vi "AlliGator Plot Histogram Event.vi"(8 "Error In":errorcluster, 11 "Mouse Click Event Data":T1) -> (0 "Error Out":errorcluster, 1 "Message":string)   [LabVIEW 2021, in "AlliGator Lifetime & Other Parameters.lvlib"]
uses:
  AlliGator Lifetime & Other Parameters.lvlib
  Graphs/XY Graph/XY Graph Mouse Click Event Data.ctl
  Graphs/XY Graph/XY Graph Refnum.ctl
  <vilib>/Utility/miscctls.llb/LVPoint32TypeDef.ctl
  AlliGator Lifetime & Other Parameters Plot Metadata.ctl
  Graphs/Get Plot at Mouse Click (XY Graph)/Get Plot at Mouse Click [AAC].vi
  Graphs/XY Graph/XY Graph Get Plots Metadata.vi
  Graphs/Graphs.lvlib
  Histograms/Histogram Window.lvlib
  Graphs/XY Graph/XY Graph Add-Ons.lvlib
panel:
  # "see the License on the block diagram (Ctrl+E or Window:Show Block Diagram)"
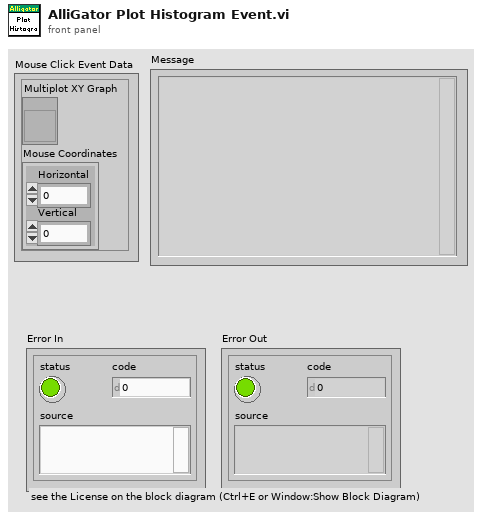
[diagram p1: front panel]
types:
  T1 = typedef "XY Graph Add-Ons.lvlib/XY Graph Mouse Click Event Data.ctl" = cluster{"Multiplot XY Graph":T2, "Mouse Coordinates":T3}
  T2 = typedef "XY Graph Add-Ons.lvlib/XY Graph Refnum.ctl" = refnum<vi>
  T3 = typedef "LVPoint32TypeDef.ctl" = cluster{"Horizontal":i32, "Vertical":i32}
  T4 = typedef "AlliGator Lifetime & Other Parameters.lvlib/AlliGator Lifetime & Other Parameters Plot Metadata.ctl" = cluster{"Intensity Array":dbl[]}
  T5 = typedef "Histogram Window.lvlib/Linear Histogram Options.ctl" = cluster{"Bin Size":dbl, "Bin Number":i32, "Bin Option":T6, "Min Value":dbl, "Max Value":dbl, "Filter NaN & Infinite Values":bool, "Frequency Plot":bool, "Align Bins":bool, "Bin Location":T7, "Project Outside Values":bool, "Max Histogram Size":i32}
  T6 = typedef "Histogram Window.lvlib/Histogram Bin Option.ctl" = enum32{"Bin Number", "Bin Size"}
  T7 = typedef "Histogram Window.lvlib/Histogram Bin Position.ctl" = enum16{"Left", "Center", "Right"}
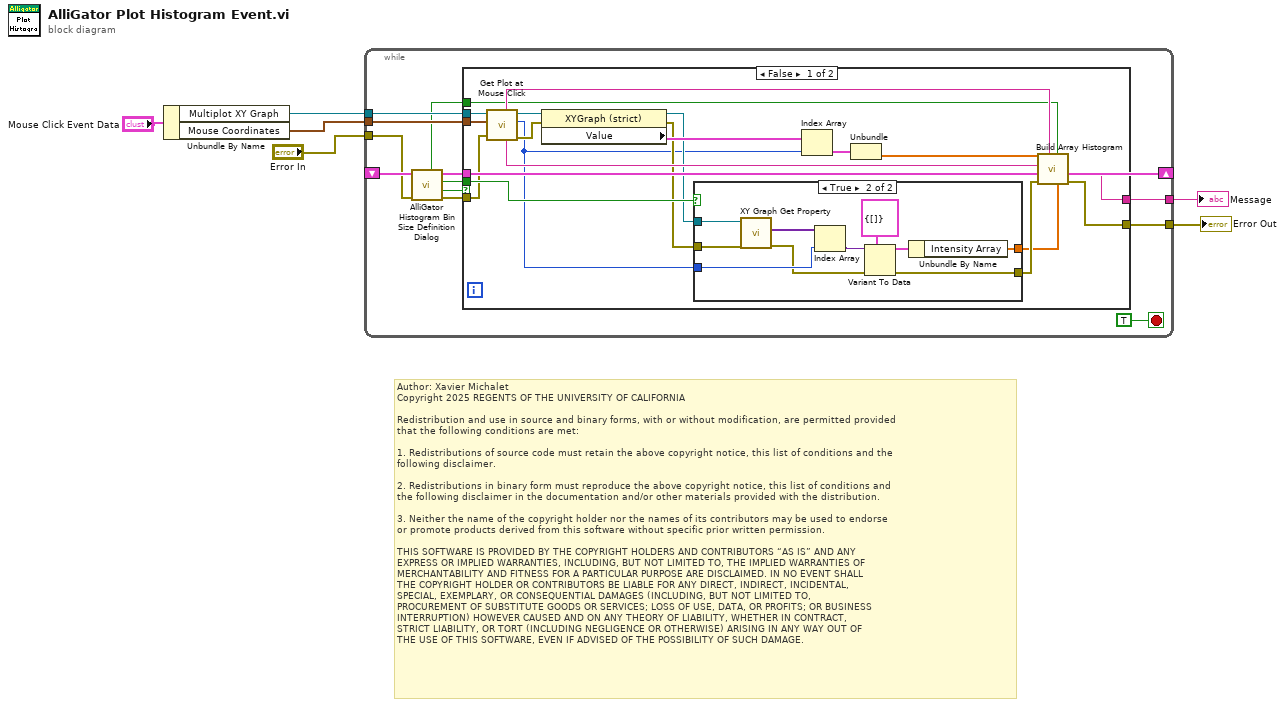
[diagram p0: block diagram]
diagram:
  # "Author: Xavier Michalet\nCopyright 2025 REGENTS OF THE UNIVERSITY OF CALIFORNIA\n\nRedistribution and use in source and binary forms, with or without modification, are permitted provided\nthat the following conditions are met:\n\n1. Redistributions of source code must retain the above copyright notice, this list of conditions and the\nfollowing disclaimer.\n\n2. Redistributions in binary form must reproduce the above copyright notice, this list of conditions and\nthe following disclaimer in the documentation and/or other materials provided with the distribution.\n\n3. Neither the name of the copyright holder nor the names of its contributors may be used to endorse \nor promote products derived from this software without specific prior written permission.\n\nTHIS SOFTWARE IS PROVIDED BY THE COPYRIGHT HOLDERS AND CONTRIBUTORS “AS IS” AND ANY \nEXPRESS OR IMPLIED WARRANTIES, INCLUDING, BUT NOT LIMITED TO, THE IMPLIED WARRANTIES OF\nMERCHANTABILITY AND FITNESS FOR A PARTICULAR PURPOSE ARE DISCLAIMED. IN NO EVENT SHALL\nTHE COPYRIGHT HOLDER OR CONTRIBUTORS BE LIABLE FOR ANY DIRECT, INDIRECT, INCIDENTAL, \nSPECIAL, EXEMPLARY, OR CONSEQUENTIAL DAMAGES (INCLUDING, BUT NOT LIMITED TO, \nPROCUREMENT OF SUBSTITUTE GOODS OR SERVICES; LOSS OF USE, DATA, OR PROFITS; OR BUSINESS\nINTERRUPTION) HOWEVER CAUSED AND ON ANY THEORY OF LIABILITY, WHETHER IN CONTRACT, \nSTRICT LIABILITY, OR TORT (INCLUDING NEGLIGENCE OR OTHERWISE) ARISING IN ANY WAY OUT OF\nTHE USE OF THIS SOFTWARE, EVEN IF ADVISED OF THE POSSIBILITY OF SUCH DAMAGE."
  n1 = Unbundle By Name("Mouse Click Event Data") -> ("Multiplot XY Graph"=w4:T2, "Mouse Coordinates"=w3:T3)
  n2 = while {
    tunnel: w4 -> [w18]
    tunnel: w3 -> [w17]
    tunnel: "Error In" -> [w10]
    shift-right: [w12] -> _
    shift-left: _ -> [w16]
    tunnel: [w9] -> w2
    tunnel: [w8] -> w1
    stop <- TRUE stop-if-true
    n3 = call "AlliGator Histogram Bin Size Definition Dialog.vi"("error in (no error)"=w10, "Histogram Options in"=w16) -> ("error out"=w11:errorcluster, "Cancelled?"=w14:bool, "Intensity-weighted Histogram (out)"=w13:bool, "Histogram Options"=w12:T5, "Normalized Weighted Histogram (out)"=w7:bool)  [unwired: 5 in]
    n4 = case shown="False" w14 {
      tunnel: w18 -> [w34 _]
      tunnel: w17 -> [w33 _]
      tunnel: w13 -> [w30 _]
      tunnel: w12 -> [w29 _]
      tunnel: w11 -> [w26 w50]
      tunnel: [w21 _] -> w9
      tunnel: [w20 w50] -> w8
      tunnel: w7 -> [w19 _]
      frame False {
        n5 = call-poly "Get Plot at Mouse Click.vi"("error in (no error)"=w26, "Mouse Click Coordinates"=w33, "XY Graph in"=w34) -> ("error out"=w37:errorcluster, "Plot at Coordinates"=w24:i32, "XY Graph out"=w38:T2, "Plot Name"=w31:string, "Graph Name"=w28:string)  [unwired: 2 in, 2 out]
        n6 = property class="XYGraph (strict)"(reference=w38, error in=w37) -> (reference out=w27:T2, error out=w25:errorcluster, "Value"=w36:cluster{"X Array":dbl[], "Y Array":dbl[]}[])
        n7 = case shown="True" w30 {
          tunnel: w25 -> [w39 w48]
          tunnel: w27 -> [_ w49]
          tunnel: w24 -> [_ w46]
          tunnel: [w39 w41] -> w23
          tunnel: [_ w40] -> w22
          frame False {
          }
          frame True {
            n8 = call-poly "XY Graph Get Property.vi"("Error In"=w48, "XYGraph Ref"=w49) -> ("Error Out"=w45:errorcluster, "Plot Metadata"=w47:variant[])  [unwired: 6 in, 2 out]
            n9 = Index Array(array=w47, index=w46) -> (element=w43:variant)
            n10 = Variant To Data(error in=w45, type=T4 {"Intensity Array"=[]} ("Array"), Variant=w43) -> (data=w42:T4, error out=w41:errorcluster)
            n11 = Unbundle By Name(w42) -> ("Intensity Array"=w40:dbl[])
          }
        }
        n12 = Index Array(array=w36, index=w24) -> (element=w35:cluster{"X Array":dbl[], "Y Array":dbl[]})
        n13 = Unbundle(w35) -> ("Y Array"=w32:dbl[])  [unwired: 1 out]
        n14 = call "Build Array Histogram.vi"("Weights"=w22, "Normalized Weighted Histogram"=w19, "Graph Caption (or Label) Text"=w28, "error in (no error)"=w23, "Histogram Options"=w29, "Plot/Dataset Name"=w31, "Array"=w32) -> ("error out"=w20:errorcluster, "Message"=w21:string)  [unwired: 2 in, 1 out]
      }
      frame True {
      }
    }
  }
  "Error Out" <- w1
  "Message" <- w2
